vi "SinusoidPattern.vi"(7 "Phase (2pi unit)":dbl, 9 "Frequency Ratio":dbl=1.0, 11 "N point":i32) -> (1 "Unit Pattern":dbl[](array[numeric]), 3 "Points":i32[](array[numeric]))   [LabVIEW 2015, in "ArbitraryFunctions.lvlib"]
uses:
  ArbitraryFunctions.lvlib
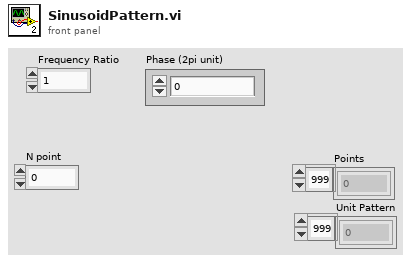
[diagram p1: front panel]
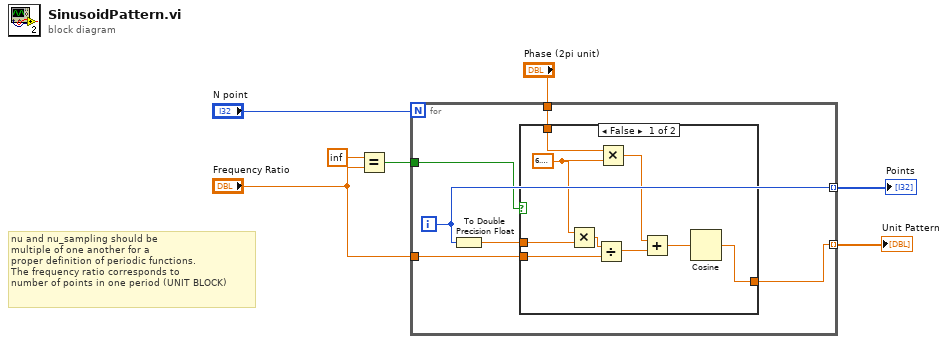
[diagram p0: block diagram]
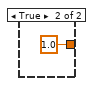
[diagram p2: hidden frame]
diagram:
  # "nu and nu_sampling should be \nmultiple of one another for a \nproper definition of periodic functions. \nThe frequency ratio corresponds to\nnumber of points in one period (UNIT BLOCK)"
  n1 = Equal?(x=inf, y="Frequency Ratio") -> (x = y?=w1:bool)
  n2 = for {
    N: "N point" -> [_]
    tunnel: [w12] -> w7 mode=indexing
    tunnel: [w10] -> w6 mode=indexing
    tunnel: "Phase (2pi unit)" -> [w11]
    tunnel: "Frequency Ratio" -> [w9]
    tunnel: w1 -> [w8]
    i -> [w12]
    n3 = To Double Precision Float(number=w12) -> (double precision float=w13:dbl)
    n4 = case shown="False" w8 {
      tunnel: w13 -> [w21 _]
      tunnel: w11 -> [w19 _]
      tunnel: [w16 1.0] -> w10
      tunnel: w9 -> [w14 _]
      frame False {
        w15 = 6.283185307179586
        n5 = Multiply(x=w15, y=w21) -> (x*y=w22:dbl)
        n6 = Divide(x=w22, y=w14) -> (x/y=w20:dbl)
        n7 = Multiply(x=w19, y=w15) -> (x*y=w18:dbl)
        n8 = Add(x=w18, y=w20) -> (x+y=w17:dbl)
        n9 = Cosine(x=w17) -> (cos(x)=w16:dbl)
      }
      frame True {
      }
    }
  }
  "Points" <- w7
  "Unit Pattern" <- w6
